vi "Insert Into SubPanel.vi"(8 "error in (no error)":errorcluster caption="Error In", 9 "SubPanel Ref":refnum<vi>, 10 "VI Path":path, 11 "VI Ref In":refnum<vi>) -> (0 "error out":errorcluster caption="Error Out")   [LabVIEW 2020]
panel:
  # "传入VI的引用或者VI路径程序都可以自动判断"
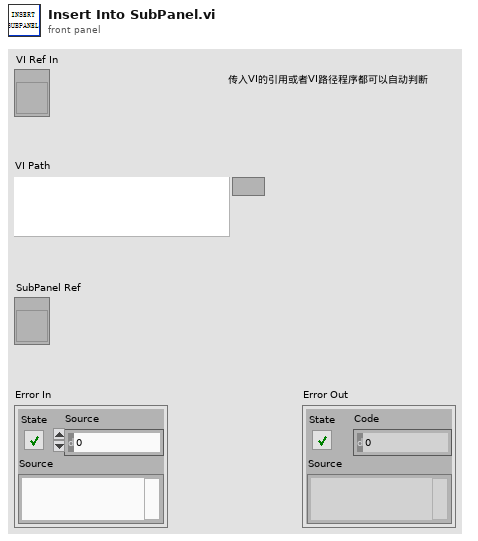
[diagram p1: front panel]
types:
  T1 = enum32{"Invalid", "Standard", "Closed", "Hidden", "Minimized", "Maximized"}
  T2 = enum32{"Bad", "Idle", "Run top level", "Running"}
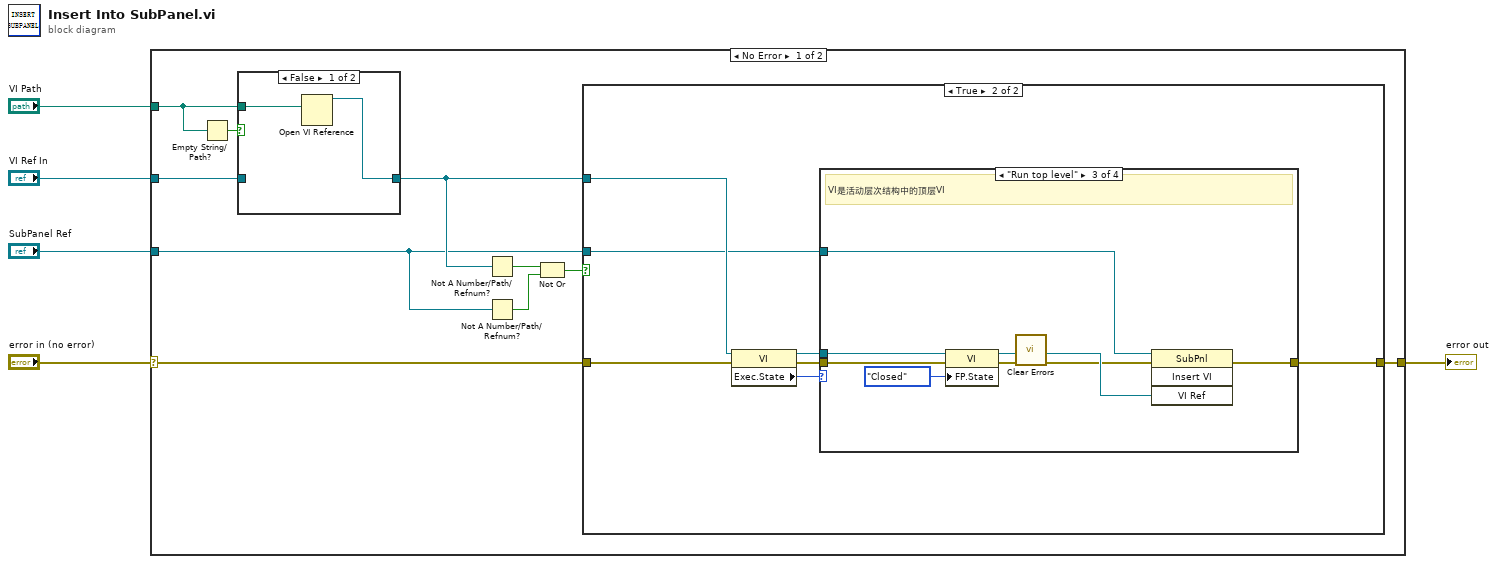
[diagram p0: block diagram]
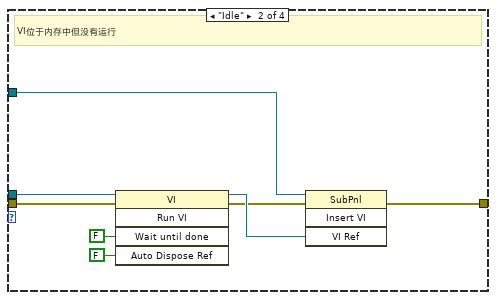
[diagram p4: hidden frame]
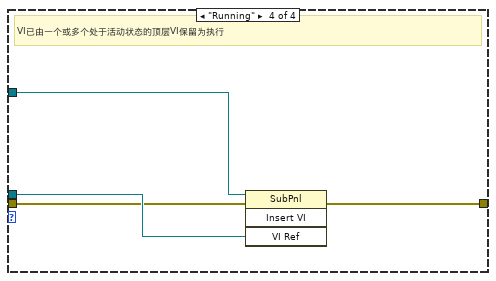
[diagram p5: hidden frame]
diagram:
  n1 = case shown="No Error" "error in (no error)" {
    selector: "error in (no error)" -> [w15 w48]
    tunnel: [w14 w48] -> w4
    tunnel: "VI Path" -> [w13 _]
    tunnel: "SubPanel Ref" -> [w9 _]
    tunnel: "VI Ref In" -> [w11 _]
    frame No Error {
      n2 = Empty String/Path?(string/path=w13) -> (empty?=w12:bool)
      n3 = case shown="False" w12 {
        tunnel: w13 -> [w46 _]
        tunnel: [w45 w47] -> w10
        tunnel: w11 -> [_ w47]
        frame False {
          n4 = Open VI Reference(vi path=w46) -> (vi reference=w45:refnum<vi>)  [unwired: 5 in, 1 out]
        }
        frame True {
        }
      }
      n5 = Not A Number/Path/Refnum?(number/path/refnum=w10) -> (NaN/Path/Refnum?=w7:bool)
      n6 = Not A Number/Path/Refnum?(number/path/refnum=w9) -> (NaN/Path/Refnum?=w8:bool)
      n7 = Not Or(1:w8, 2:w7) -> (0:w6:bool)
      n8 = case shown="True" w6 {
        tunnel: w15 -> [w16 w23]
        tunnel: [w16 w22] -> w14
        tunnel: w9 -> [_ w20]
        tunnel: w10 -> [_ w21]
        frame False {
        }
        frame True {
          n9 = property class="VI"(reference=w21, error in=w23) -> (reference out=w18:refnum<vi>, error out=w17:errorcluster, "Exec.State"=w19:T2)
          n10 = case shown="\"Run top level\"" w19 {
            tunnel: w18 -> [_ w32 w40 w43]
            tunnel: w20 -> [_ w29 w38 w44]
            tunnel: w17 -> [w24 w27 w34 w42]
            tunnel: [w24 w25 w36 w41] -> w22
            frame "Bad", Default {
              # "VI包含错误并且无法执行。"
            }
            frame "Idle" {
              # "VI位于内存中但没有运行"
              n11 = invoke class="VI" method="Run VI"(reference=w32, error in=w27, "Wait until done"=FALSE ("结束前等待"), "Auto Dispose Ref"=FALSE ("自动销毁引用")) -> (reference out=w28:refnum<vi>, error out=w26:errorcluster)  [unwired: 1 in, 3 out]
              n12 = invoke class="SubPnl" method="Insert VI"(reference=w29, error in=w26, "VI Ref"=w28) -> (error out=w25:errorcluster)  [unwired: 1 in, 3 out]
            }
            frame "Run top level" {
              # "VI是活动层次结构中的顶层VI"
              n13 = property class="VI"(reference=w40, error in=w34, "FP.State"=T1."Closed" ("前面板窗口:状态")) -> (reference out=w37:refnum<vi>, error out=w35:errorcluster)
              n14 = call <vilib>:"Clear Errors.vi"("error in (no error)"=w35) -> ("error out"=w33:errorcluster)  [unwired: 5 in, 1 out]
              n15 = invoke class="SubPnl" method="Insert VI"(reference=w38, error in=w33, "VI Ref"=w37) -> (error out=w36:errorcluster)  [unwired: 1 in, 3 out]
            }
            frame "Running" {
              # "VI已由一个或多个处于活动状态的顶层VI保留为执行"
              n16 = invoke class="SubPnl" method="Insert VI"(reference=w44, error in=w42, "VI Ref"=w43) -> (error out=w41:errorcluster)  [unwired: 1 in, 3 out]
            }
          }
        }
      }
    }
    frame Error {
    }
  }
  "error out" <- w4
